vi "Get Class Path from Class Name.vi"(8 "error in (no error)":errorcluster, 9 "Class Name":string, 10 "TestProjectClasses":path[](array[path]), 11 "Test Project":path) -> (0 "error out":errorcluster, 1 "Class Path":path)   [LabVIEW 2011, in "GraphicalTestRunner.lvlib"]
uses:
  GraphicalTestRunner.lvlib
  <userlib>/_OpenG.lib/file/file.llb/Strip Path Extension - Path__ogtk.vi
  <userlib>/_OpenG.lib/file/file.llb/Strip Path Extension - String__ogtk.vi
  <userlib>/_OpenG.lib/file/file.llb/Strip Path - Arrays__ogtk.vi
  <userlib>/_OpenG.lib/file/file.llb/Strip Path Extension - 1D Array of Strings__ogtk.vi
  <userlib>/_OpenG.lib/file/file.llb/Strip Path Extension - 1D Array of Paths__ogtk.vi
panel:
  # "Copyright © 2007 James Kring, Inc. All rights reserved.\n\nAuthor: Omar Mussa [omar.mussa@jameskring.com]\n\nThis library is provided \"AS IS\" ,WITHOUT WARRANTIES OR \nCONDITIONS OF ANY KIND, either express or implied.\n\nJames Kring, Inc. -- http://www.jameskring.com"
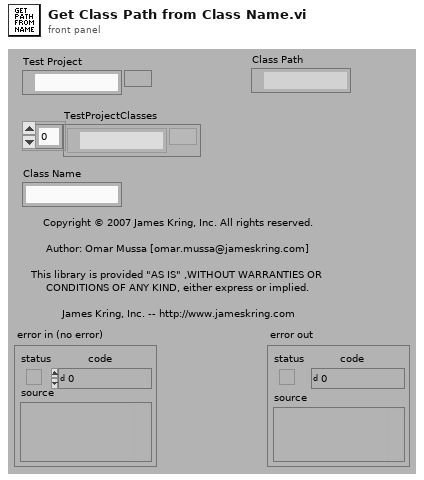
[diagram p1: front panel]
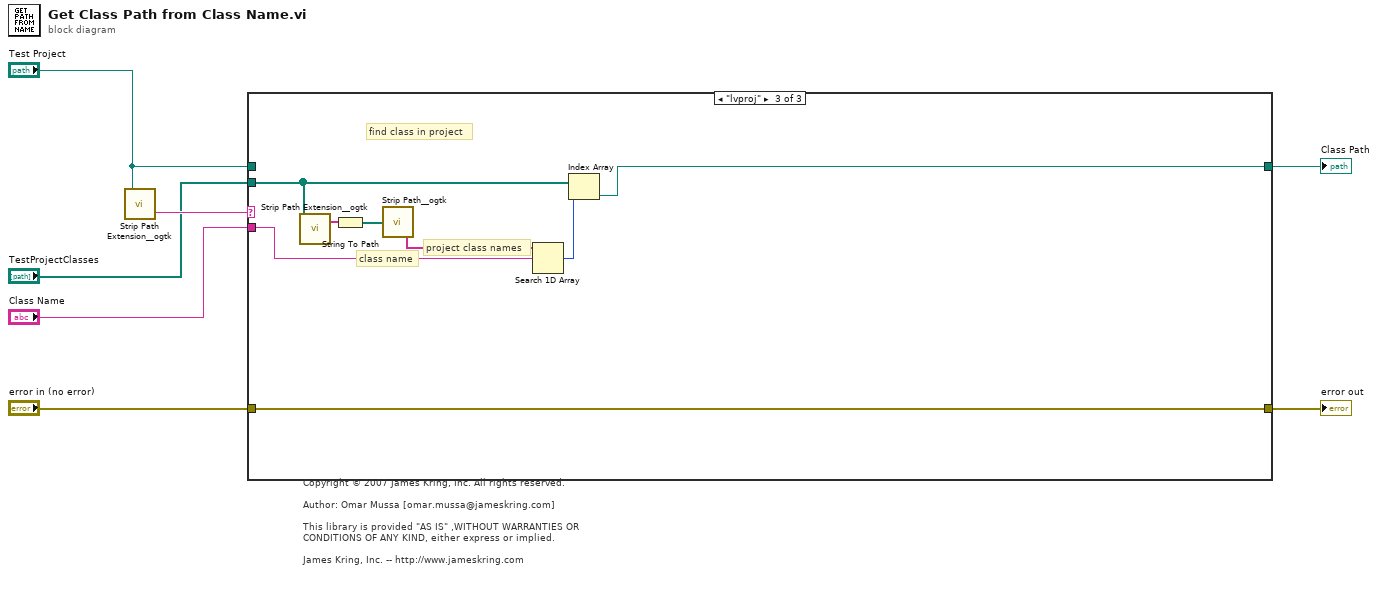
[diagram p0: block diagram]
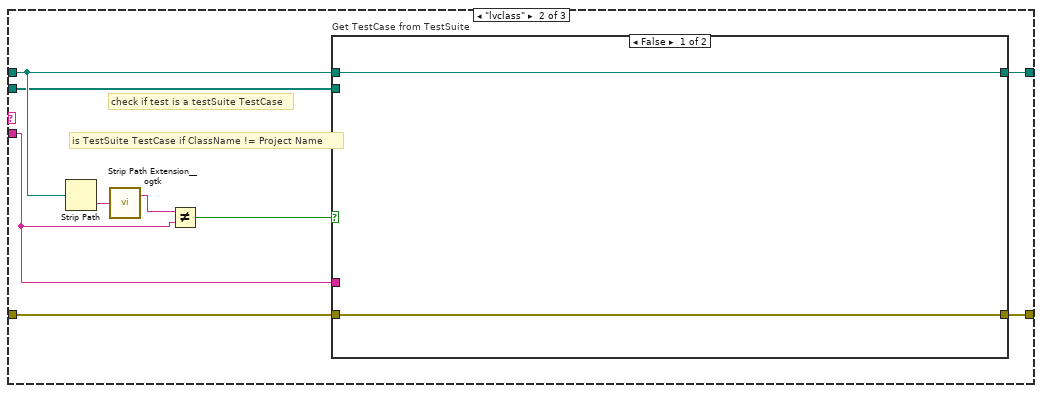
[diagram p3: hidden frame]
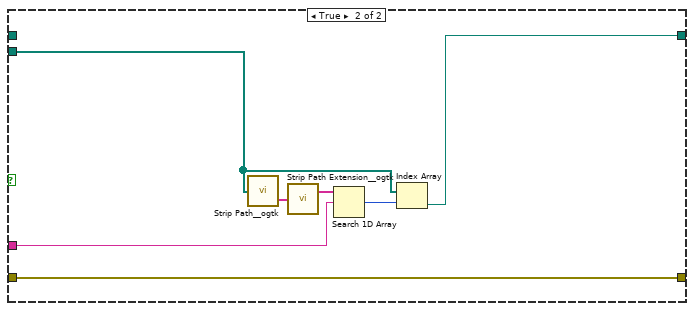
[diagram p4: hidden frame]
diagram:
  # "Copyright © 2007 James Kring, Inc. All rights reserved.\n\nAuthor: Omar Mussa [omar.mussa@jameskring.com]\n\nThis library is provided \"AS IS\" ,WITHOUT WARRANTIES OR \nCONDITIONS OF ANY KIND, either express or implied.\n\nJames Kring, Inc. -- http://www.jameskring.com"
  n1 = call-poly <userlib>:"Strip Path Extension__ogtk.vi"("path"="Test Project") -> ("extension"=w5:string)  [unwired: 1 out]
  n2 = case shown="\"lvproj\"" w5 {
    tunnel: [w9 w16 w30] -> w7
    tunnel: "Test Project" -> [w9 w15 _]
    tunnel: "Class Name" -> [_ w14 w28]
    tunnel: "TestProjectClasses" -> [_ w10 w31]
    tunnel: "error in (no error)" -> [w8 w12 w29]
    tunnel: [w8 w11 w29] -> w1
    frame Default {
    }
    frame "lvclass" {
      # "is TestSuite TestCase if ClassName != Project Name"
      # "check if test is a testSuite TestCase"
      n3 = Strip Path(path=w15) -> (name=w18:string)  [unwired: 1 out]
      n4 = call-poly <userlib>:"Strip Path Extension__ogtk.vi"("path"=w18) -> ("root"=w13:string)  [unwired: 1 out]
      n5 = Not Equal?(x=w13, y=w14) -> (x != y?=w17:bool)
      n6 = case "Get TestCase from TestSuite" shown="False" w17 {
        tunnel: [w20 w23] -> w16
        tunnel: w15 -> [w20 _]
        tunnel: w14 -> [_ w26]
        tunnel: w12 -> [w19 w21]
        tunnel: [w19 w21] -> w11
        tunnel: w10 -> [_ w22]
        frame False {
        }
        frame True {
          n7 = call-poly <userlib>:"Strip Path__ogtk.vi"("path"=w22) -> ("name"=w25:string[])  [unwired: 1 out]
          n8 = call-poly <userlib>:"Strip Path Extension__ogtk.vi"("paths"=w25) -> ("roots"=w27:string[])  [unwired: 1 out]
          n9 = Search 1D Array(1D array=w27, element=w26) -> (index of element=w24:i32)  [unwired: 1 in]
          n10 = Index Array(array=w22, index=w24) -> (element=w23:path)
        }
      }
    }
    frame "lvproj" {
      # "class name"
      # "project class names"
      # "find class in project"
      n11 = call-poly <userlib>:"Strip Path Extension__ogtk.vi"("paths"=w31) -> ("roots"=w35:string[])  [unwired: 1 out]
      n12 = String To Path(string=w35) -> (path=w34:path[])
      n13 = call-poly <userlib>:"Strip Path__ogtk.vi"("path"=w34) -> ("name"=w33:string[])  [unwired: 1 out]
      n14 = Search 1D Array(1D array=w33, element=w28) -> (index of element=w32:i32)  [unwired: 1 in]
      n15 = Index Array(array=w31, index=w32) -> (element=w30:path)
    }
  }
  "Class Path" <- w7
  "error out" <- w1
